vi "FRCts20_EspEngine_ConvertToComment.vi"(8 "error in (no error)":errorcluster, 10 "Comment":T1) -> (0 "error out":errorcluster, 2 "Comment":T2)   [LabVIEW 2014, in "FRCts20_EspEngine.lvlib"]
uses:
  FRCts20_EspEngine.lvlib
  TypeDefs/FRCts20_EspEngine_Comment.ctl
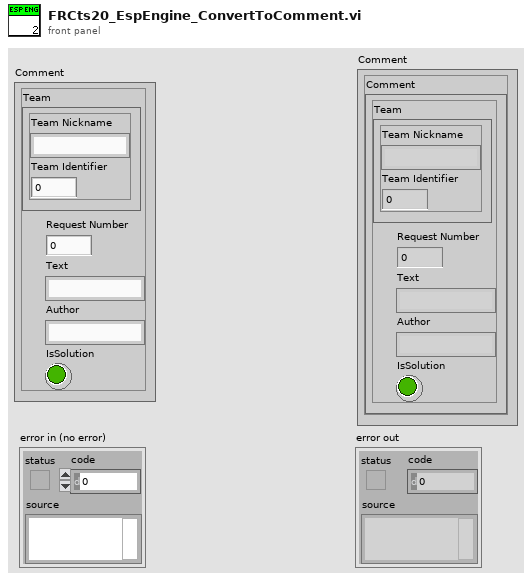
[diagram p1: front panel]
types:
  T1 = cluster{"Request Number":dbl, "Text":string, "Author":string, "IsSolution":bool, "Team":cluster{"Team Nickname":string, "Team Identifier ":dbl}}
  T2 = typedef "FRCts20_EspEngine.lvlib/FRCts20_EspEngine_Comment.ctl" = cluster{"Comment":cluster{"Request Number":dbl, "Text":string, "Author":string, "IsSolution":bool, "Team":cluster{"Team Nickname":string, "Team Identifier ":dbl}}}
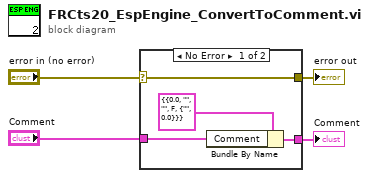
[diagram p0: block diagram]
diagram:
  n1 = case shown="No Error" "error in (no error)" {
    selector: "error in (no error)" -> [w5 w9]
    tunnel: [w5 w9] -> w4
    tunnel: "Comment" -> [w6 _]
    tunnel: [w7 _] -> w1
    frame No Error {
      n2 = Bundle By Name(cluster=T2 {"Comment"={"Request Number"=0.0, "Text"="", "Author"="", "IsSolution"=FALSE, "Team"={"Team Nickname"="", "Team Identifier "=0.0}}} ("Comment"), "Comment"=w6) -> (w7:T2)
    }
    frame Error {
    }
  }
  "Comment" <- w1
  "error out" <- w4
